vi "Absolute Value.vi"   [LabVIEW 2017, in "NI_Matrix.lvlib"]
doc: "Returns the absolute value of the input."
uses:
  <vilib>/Analysis/Matrix/NI_Matrix.lvlib
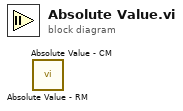
[diagram p0: block diagram]
diagram:
  n1 = call <vilib>:"Absolute Value - RM.vi"() -> ()  [unwired: 1 in, 1 out]
  n2 = call <vilib>:"Absolute Value - CM.vi"() -> ()  [unwired: 1 in, 1 out]
